vi "Select Class.vi"(7 "Instrument":T1, 8 "error in":errorcluster, 11 "Class Path":path=path "C:/GitHub/OOP Template/HAL/Concrete") -> (0 "error out":errorcluster, 3 "Class Ref":refnum<class>)   [LabVIEW 2019, in "Measuremtn Abstraction.lvlib"]
uses:
  Measuremtn Abstraction.lvlib
  Controls/Instrument -Enum.ctl
  Hardware Abstraction/Harware Abstraction/DIO/DIO.lvclass
  C:/Workspace/gip-fct/Sequence/CodeModules/Hardware Abstraction/Harware Abstraction/Instrument/Instrument.lvclass
  Hardware Abstraction/Harware Abstraction/Switch/Switch.lvclass
  Hardware Abstraction/Harware Abstraction/MultiIO/MIO.lvclass
  Hardware Abstraction/Harware Abstraction/Analog out/Analog out.lvclass
  Hardware Abstraction/Harware Abstraction/Instrument/Instrument.lvclass
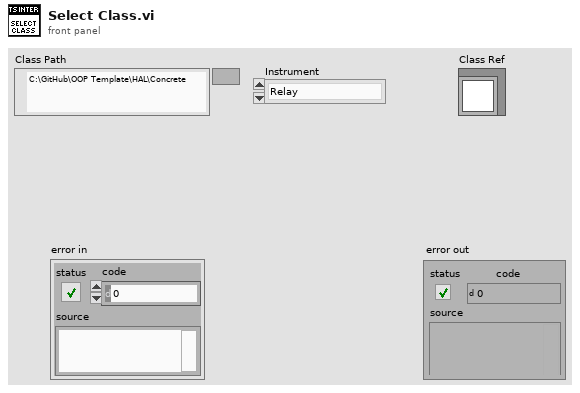
[diagram p1: front panel]
types:
  T1 = typedef "Measuremtn Abstraction.lvlib/Instrument -Enum.ctl" = enum16{"Relay", "MUX", "DMM", "DCPS", "ACPS"}
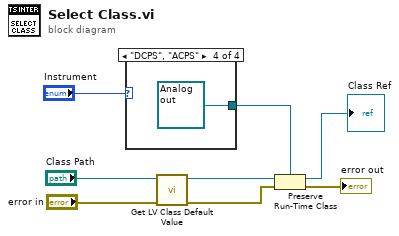
[diagram p0: block diagram]
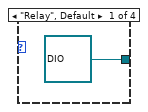
[diagram p2: hidden frame]
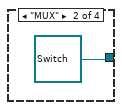
[diagram p3: hidden frame]
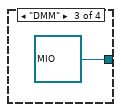
[diagram p4: hidden frame]
diagram:
  n1 = case shown="\"DCPS\", \"ACPS\"" "Instrument" {
    tunnel: [refnum<class "DIO.lvclass"> refnum ("Hardware Abstration.lvlib:DIO.lvclass") refnum<class "Switch.lvclass"> refnum ("Hardware Abstration.lvlib:Switch.lvclass") refnum<class "MIO.lvclass"> refnum ("Hardware Abstration.lvlib:MIO.lvclass") refnum<class "Analog out.lvclass"> refnum ("Hardware Abstration.lvlib:Analog out.lvclass")] -> w2
    frame "Relay", Default {
    }
    frame "MUX" {
    }
    frame "DMM" {
    }
    frame "DCPS", "ACPS" {
    }
  }
  n2 = call <vilib>:"Get LV Class Default Value.vi"("error in (no error)"="error in", "class path"="Class Path") -> ("error out"=w7:errorcluster, "object"=w3:refnum<class>)  [unwired: 8 in]
  n3 = Preserve Run-Time Class(object in=w3, error in=w7, 2:w2) -> (object out=→"Class Ref":refnum<class "Instrument.lvclass">, error out=→"error out":errorcluster)
